vi "OE1022D_Configure Sine Out Channel B.vi"(0 "VISA resource name":refnum<visa-resource-name>, 1 "Start Value(V)":sgl=1.0 format="%.3f", 2 "Stop Valve(V)":sgl=5.0 format="%.3f", 3 "Step Time(ms)":sgl=1000.0, 5 "SineOut Mode":u8(ring) items=["Fixed", "Linear", "Log"], 9 "Sine Output Amplitude (V)":sgl=1.0 format="%.3f", 11 "error in (no error)":errorcluster, 12 "Sine Step Valve(V)":sgl=1.0 format="%.3f", 13 "Sine Step Percent(%)":sgl=10.0 format="%.3f", 14 "Sine Run Mode":u8(ring) items=["Stop", "Single", "Loop"]) -> (4 "VISA resource name out":refnum<visa-resource-name>, 15 "error out":errorcluster)   [LabVIEW 2021]
doc: "Configures the reference source and the internal oscillator."
panel:
  out "结果字符串":string
  # "Signal Generator"
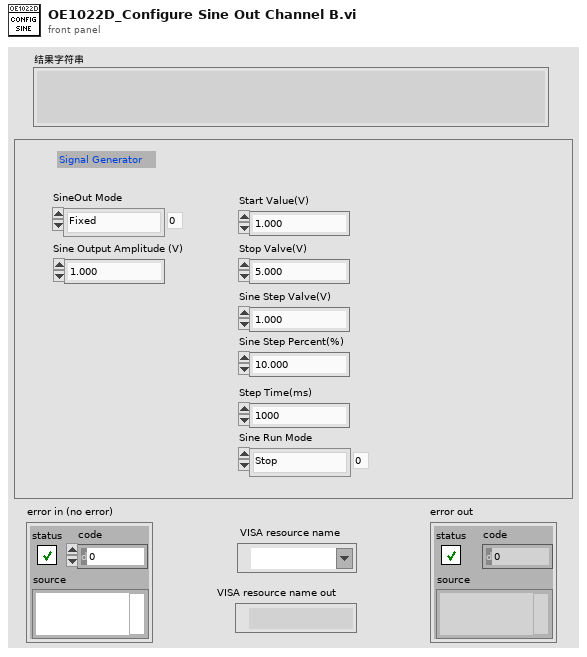
[diagram p1: front panel]
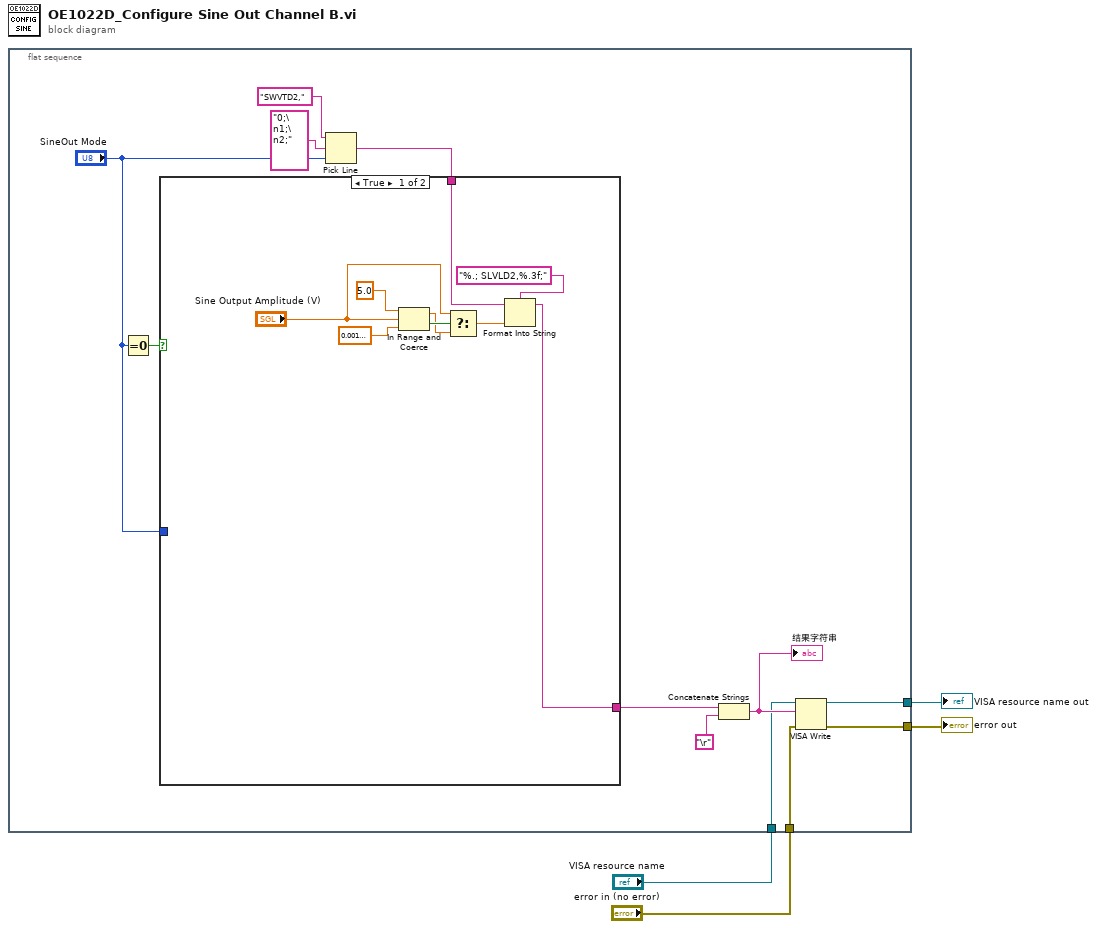
[diagram p0: block diagram]
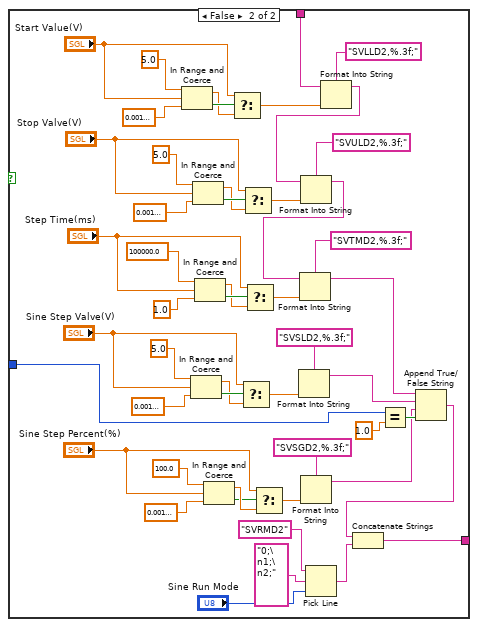
[diagram p2: hidden frame]
diagram:
  n1 = flat-sequence {
    tunnel: "error in (no error)" -> [w13]
    tunnel: "VISA resource name" -> [w14]
    tunnel: [w7] -> w2
    tunnel: [w6] -> w1
    frame #0 {
      n2 = Equal To 0?(x="SineOut Mode") -> (x = 0?=w10:bool)
      n3 = Pick Line(string ("")="SWVTD2,", multi-line string="0;\n1;\n2;", line index="SineOut Mode") -> (output string=w5:string)
      n4 = case shown="True" w10 {
        tunnel: w5 -> [w19 w62]
        tunnel: "SineOut Mode" -> [_ w33]
        tunnel: [w18 w29] -> w8
        frame True {
          n5 = In Range and Coerce(upper limit=sgl 5.0 ("上限"), x="Sine Output Amplitude (V)", lower limit=sgl 0.001 ("下限")) -> (coerced(x)=w17:sgl, In Range?=w23:bool)
          n6 = Select(t="Sine Output Amplitude (V)", s=w23, f=w17) -> (s? t:f=w25:sgl)
          n7 = Format Into String(format string="%.; SLVLD2,%.3f;", initial string=w19, w25) -> (resulting string=w18:string)  [unwired: 1 in, 1 out]
        }
        frame False {
          n8 = In Range and Coerce(upper limit=sgl 5.0 ("上限"), x="Start Value(V)", lower limit=sgl 0.001 ("下限")) -> (coerced(x)=w69:sgl, In Range?=w73:bool)
          n9 = In Range and Coerce(upper limit=sgl 5.0 ("上限"), x="Sine Step Valve(V)", lower limit=sgl 0.001 ("下限")) -> (coerced(x)=w27:sgl, In Range?=w59:bool)
          n10 = In Range and Coerce(upper limit=sgl 5.0 ("上限"), x="Stop Valve(V)", lower limit=sgl 0.001 ("下限")) -> (coerced(x)=w28:sgl, In Range?=w66:bool)
          n11 = In Range and Coerce(upper limit=sgl 100000.0 ("上限"), x="Step Time(ms)", lower limit=sgl 1.0 ("下限")) -> (coerced(x)=w50:sgl, In Range?=w53:bool)
          n12 = In Range and Coerce(upper limit=sgl 100.0 ("上限"), x="Sine Step Percent(%)", lower limit=sgl 0.001 ("下限")) -> (coerced(x)=w47:sgl, In Range?=w44:bool)
          n13 = Select(t="Start Value(V)", s=w73, f=w69) -> (s? t:f=w75:sgl)
          n14 = Select(t="Sine Step Valve(V)", s=w59, f=w27) -> (s? t:f=w57:sgl)
          n15 = Select(t="Stop Valve(V)", s=w66, f=w28) -> (s? t:f=w68:sgl)
          n16 = Select(t="Step Time(ms)", s=w53, f=w50) -> (s? t:f=w55:sgl)
          n17 = Select(t="Sine Step Percent(%)", s=w44, f=w47) -> (s? t:f=w42:sgl)
          n18 = Format Into String(format string="SVSLD2,%.3f;", w57) -> (resulting string=w32:string)  [unwired: 2 in, 1 out]
          n19 = Format Into String(format string="SVSGD2,%.3f;", w42) -> (resulting string=w31:string)  [unwired: 2 in, 1 out]
          n20 = Pick Line(string ("")="SVRMD2", multi-line string="0;\n1;\n2;", line index="Sine Run Mode") -> (output string=w37:string)
          n21 = Format Into String(format string="SVLLD2,%.3f;", initial string=w62, w75) -> (resulting string=w63:string)  [unwired: 1 in, 1 out]
          n22 = Format Into String(format string="SVULD2,%.3f;", initial string=w63, w68) -> (resulting string=w48:string)  [unwired: 1 in, 1 out]
          n23 = Format Into String(format string="SVTMD2,%.3f;", initial string=w48, w55) -> (resulting string=w36:string)  [unwired: 1 in, 1 out]
          n24 = Equal?(x=w33, y=1.0) -> (x = y?=w35:bool)
          n25 = Append True/False String(1:w35, 2:w31, 3:w32, 4:w36) -> (0:w30:string)
          n26 = Concatenate Strings(w30, w37) -> (w29:string)
        }
      }
      n27 = Concatenate Strings(w8, "\r") -> (w15:string)
      "结果字符串" <- w15
      n28 = VISA Write(VISA resource name=w14, write buffer=w15, error in (no error)=w13) -> (VISA resource name out=w7:refnum<visa-resource-name>, error out=w6:errorcluster)  [unwired: 1 out]
    }
  }
  "error out" <- w1
  "VISA resource name out" <- w2
